vi "Coax cable compensation.vi"(1 "TDCHits":T1[](array[typedef])) -> (0 "TDCHits Coax Compensated":T1[](array[typedef]))   [LabVIEW 2016]
uses:
  HPTDC Driver Library Folder/Library files/Typedefs/TDCHit.ctl
  Global Variables/Global Resolution.vi
  HPTDC Driver Library Folder/HPTDC Driver Library.lvlib
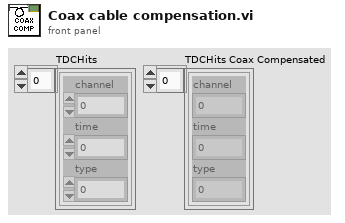
[diagram p1: front panel]
types:
  T1 = typedef "HPTDC Driver Library.lvlib/TDCHit.ctl" = cluster{"channel":u8, "time":u64, "type":u8}
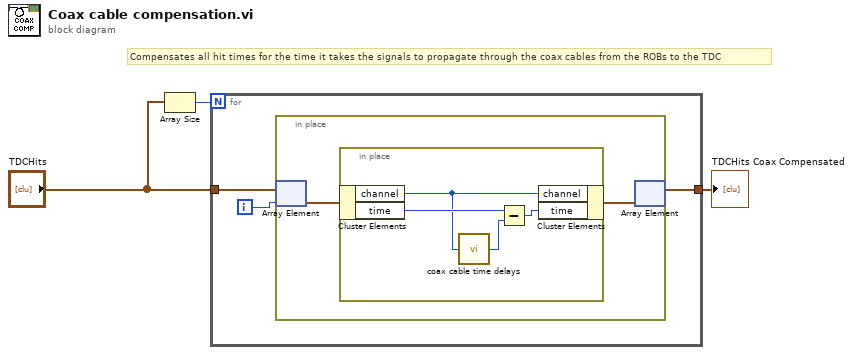
[diagram p0: block diagram]
diagram:
  # "Compensates all hit times for the time it takes the signals to propagate through the coax cables from the ROBs to the TDC"
  n1 = Array Size(array="TDCHits") -> (size(s)=w3:i32)
  n2 = for {
    N: w3 -> [_]
    tunnel: "TDCHits" -> [w6]
    tunnel: [w4] -> w1
    i -> [w5]
    n3 = in-place {
      n4 = in-place-array #1(w6, w5) -> (w8:T1)
      n5 = in-place {
        n6 = in-place-cluster #2(w8) -> ("channel"=w11:u8, "time"=w12:u64)
        n7 = call "coax cable time delays.vi"("channel"=w11) -> ("Coax cable time (x32ps)"=w10:u64)
        n8 = Subtract(x=w12, y=w10) -> (x-y=w9:u64)
        n9 = in-place-cluster #2("channel"=w11, "time"=w9) -> (w7:T1)
      }
      n10 = in-place-array #1(w7) -> (w4:T1[])  [unwired: 1 out]
    }
  }
  "TDCHits Coax Compensated" <- w1
